vi "NI_SAT_TEST_20150519_EXP_V2.vi"() -> ()   [LabVIEW 2013]
uses:
  <instrlib>/niFgen/niFgen.llb/niFgen Waveform Type.ctl
  <instrlib>/niFgen/niFgen.llb/niFgen Output Impedance.ctl
  <vilib>/Waveform/WDTOps.llb/WDT Append Waveforms DBL.vi
panel:
  out "Tabs 1 Through # Used":i32
  in  "Tab Control 3":T1(tab)
  out "Tab Control 2":T1(tab)
  out "Waveform Graph 1":waveform(dbl)(graph)
  out "Waveform Graph 2":waveform(dbl)(graph)
  out "Waveform Graph 3":waveform(dbl)(graph)
  out "Waveform Graph 4":waveform(dbl)(graph)
  out "Waveform Graph 5":waveform(dbl)(graph)
  out "Waveform Graph 6":waveform(dbl)(graph)
  out "Waveform Graph 7":waveform(dbl)(graph)
  out "Waveform Graph 8":waveform(dbl)(graph)
  out "Waveform Graph 9":waveform(dbl)(graph)
  out "Waveform Graph 10":waveform(dbl)(graph)
  out "Waveform Graph 11":waveform(dbl)(graph)
  out "Waveform Graph 12":waveform(dbl)(graph)
  out "Waveform Graph 13":waveform(dbl)(graph)
  out "Waveform Graph 14":waveform(dbl)(graph)
  out "Waveform Graph 15":waveform(dbl)(graph)
  out "Waveform Graph 16":waveform(dbl)(graph)
  out "Waveform Graph 17":waveform(dbl)(graph)
  out "Waveform Graph 18":waveform(dbl)(graph)
  out "Waveform Graph 19":waveform(dbl)(graph)
  out "Waveform Graph 20":waveform(dbl)(graph)
  out "Diff in Methods before call DMM vi and before read Wave Data (SEC)":dbl
  out "Total Elapsed Time (ms)":u32
  out "TotalElapsed Time (Sec)":dbl
  out "Waveform Graph":waveform(dbl)(graph)
  in  "Output Voltage Division":i32
  in  "Highest Output Voltage [Volts]":i32 min=-200 max=200 step=20
  in  "Rate":dbl=10.0 caption="Rate (Samples/Sec)" format="%.2f"
  in  "Waveform Points":i32=101 caption="Samples"
  in  "Function Generator Name":refnum<k15>="PXI1Slot2"
  # "Please Enter Output Voltage\nwith the desired sign. Be it positive\nor negative. Program will divide 200 and then negate, due to gain of 200 and inversion of input by amplifier"
  # "ENJOY PETER, still could use tweeking to make it run smoother and prevent more user error. Good Morning"
  # "DO NOT RAISE ABOVE 600V on TELFON MASK!!!!!!\nDO NOT RAISE ABOVE 400V on REGULAR MASK!!!"
  # "Output voltage comes from the VOLTAGE MONITOR (VM) from the amplifier with (1V VM/200V AMP)"
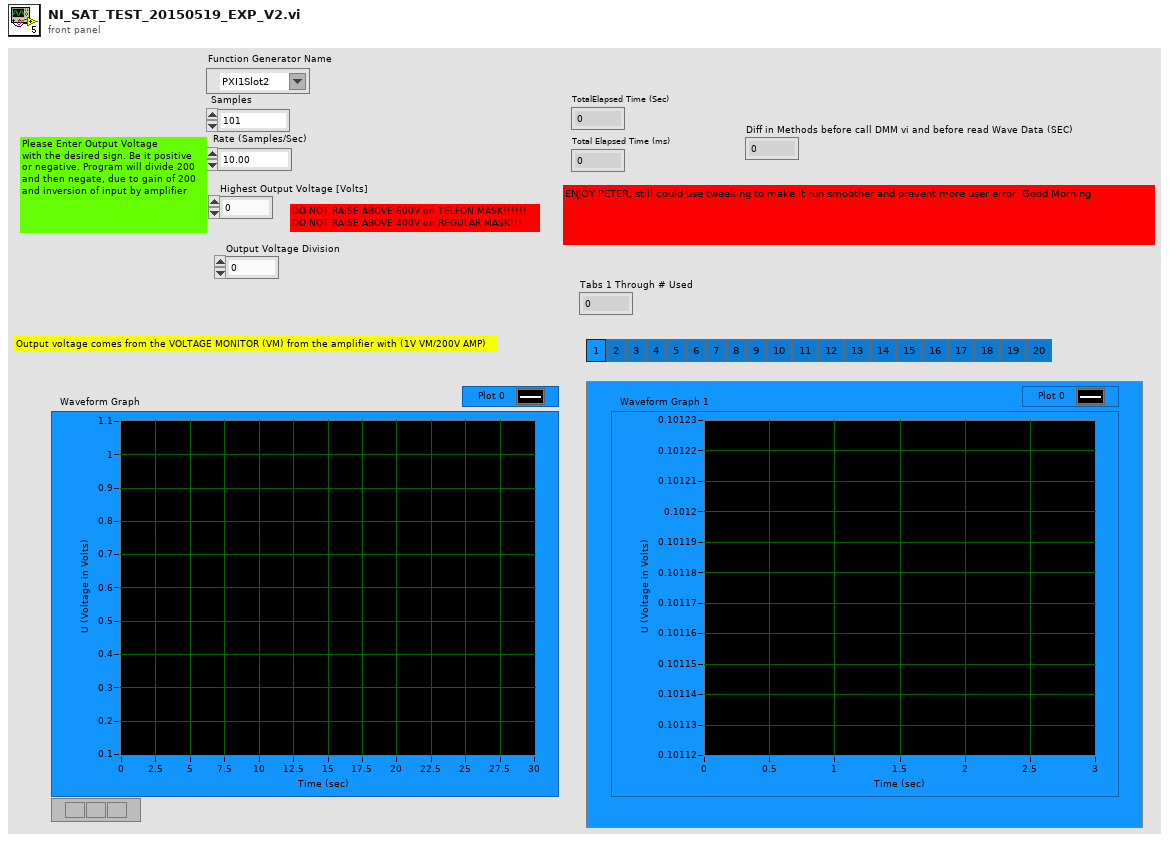
[diagram p1: front panel]
types:
  T1 = enum32{"1", "2", "3", "4", "5", "6", "7", "8", "9", "10", "11", "12", "13", "14", "15", "16", "17", "18", "19", "20"}
  T2 = enum16{"open", "replace", "create", "open or create", "replace or create", "replace or create with confirmation"}
  T3 = typedef "niFgen Output Impedance.ctl" = i32
  T4 = typedef "niFgen Waveform Type.ctl" = i32
  T5 = cluster{"channel name":string, "waveform":T4, "frequency":dbl, "amplitude":dbl, "start phase":dbl, "y":dbl, "duty cycle high":dbl, "impedance":T3, "load impedance":dbl}
  T6 = cluster{"channel name":string, "waveform":T4, "frequency":dbl, "amplitude":dbl, "start phase":dbl, "y":dbl, "duty cycle high":dbl, "impedance":T3, "load impedance":dbl}[]
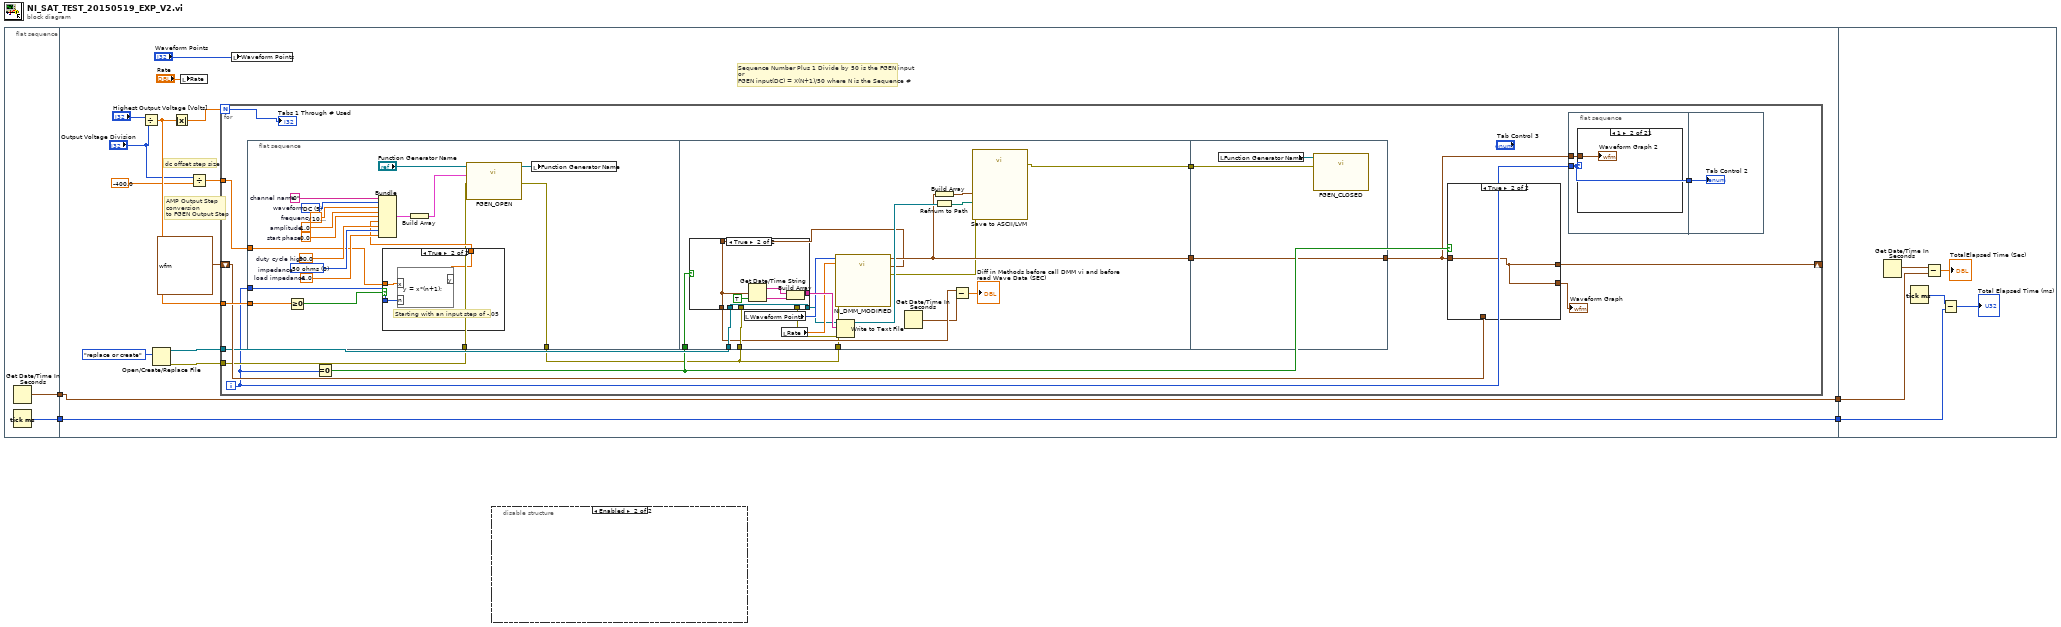
[diagram p0: block diagram]
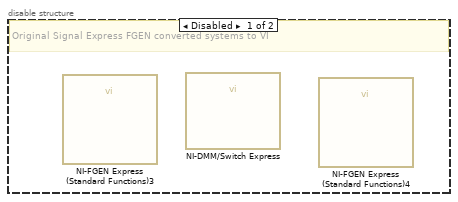
[diagram p2: hidden frame]
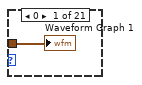
[diagram p3: hidden frame]
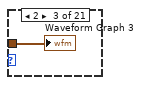
[diagram p4: hidden frame]
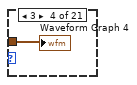
[diagram p5: hidden frame]
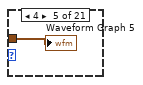
[diagram p6: hidden frame]
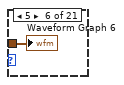
[diagram p7: hidden frame]
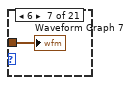
[diagram p8: hidden frame]
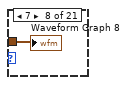
[diagram p9: hidden frame]
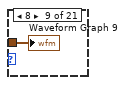
[diagram p10: hidden frame]
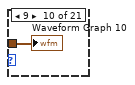
[diagram p11: hidden frame]
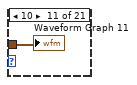
[diagram p12: hidden frame]
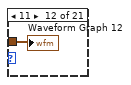
[diagram p13: hidden frame]
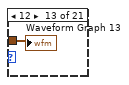
[diagram p14: hidden frame]
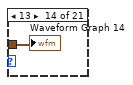
[diagram p15: hidden frame]
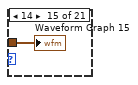
[diagram p16: hidden frame]
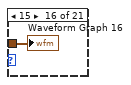
[diagram p17: hidden frame]
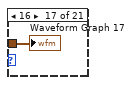
[diagram p18: hidden frame]
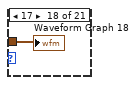
[diagram p19: hidden frame]
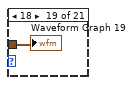
[diagram p20: hidden frame]
diagram:
  n1 = flat-sequence {
    tunnel: [w6] -> w4
    tunnel: [w5] -> w3
    tunnel: w4 -> [w12]
    tunnel: w3 -> [w11]
    tunnel: [w12] -> w2
    tunnel: [w11] -> w1
    tunnel: w2 -> [w129]
    tunnel: w1 -> [w128]
    frame #0 {
      n2 = Get Date/Time In Seconds() -> (seconds since 1Jan1904=w6:timestamp)
      n3 = Tick Count (ms)() -> (millisecond timer value=w5:u32)
    }
    frame #1 {
      # "AMP Output Step\nconversion\nto FGEN Output Step"
      # "dc offset step size"
      # "Sequence Number Plus 1 Divide by 50 is the FGEN input\nor\nFGEN input(DC) = X(N+1)/50 where N is the Sequence #"
      n4 = Divide(x="Highest Output Voltage [Volts]", y="Output Voltage Division") -> (x/y=w10:dbl)
      n5 = Open/Create/Replace File(operation (0:open)=T2."replace or create") -> (refnum out=w20:refnum<file>, error out=w19:errorcluster)  [unwired: 5 in, 1 out]
      n6 = Absolute Value(x=w10) -> (abs(x)=w14:dbl)
      n7 = local write "Rate"("Rate") -> ()
      n8 = Divide(x="Output Voltage Division", y=-400.0) -> (x/y=w9:dbl)
      n9 = for {
        N: w14 -> [w23]
        tunnel: w20 -> [w31]
        tunnel: w19 -> [w28]
        tunnel: w10 -> [w34]
        shift-right: [w26] -> _
        shift-left: waveform(dbl) {"t0"=timestamp(0 s since 1904-01-01), "dt"=1.0, "Y"=[]} ("Waveform Data") -> [w33]
        tunnel: w9 -> [w21]
        i -> [w24]
        n10 = flat-sequence {
          tunnel: w24 -> [w71]
          tunnel: w34 -> [w68]
          tunnel: w28 -> [w65]
          tunnel: [w64] -> w27
          tunnel: w21 -> [w63]
          tunnel: [w102] -> w35
          tunnel: w30 -> [w99]
          tunnel: w31 -> [w98]
          tunnel: w27 -> [w96]
          tunnel: [w93] -> w29
          tunnel: w27 -> [w89]
          tunnel: w35 -> [w126]
          tunnel: [w126] -> w25
          tunnel: w29 -> [w125]
          frame #0 {
            w72 = -1.0  # load impedance
            w73 = T3 0 items=["50 ohms", "75 ohms", "1 mega ohm"]  # impedance
            w74 = 50.0  # duty cycle high
            w75 = 0.0  # start phase
            w76 = 1.0  # amplitude
            w77 = 1000000.0  # frequency
            w78 = T4 5 items=["Sine", "Square", "Triangle", "Ramp Up", "Ramp Down", "DC", "Noise", "User"]  # waveform
            w79 = "0"  # channel name
            n11 = Greater Or Equal To 0?(x=w68) -> (x >= 0?=w67:bool)
            n12 = case shown="True" w67 {
              tunnel: w71 -> [w83 w87]
              tunnel: w63 -> [w84 w86]
              tunnel: [w82 w85] -> w66
              frame False {
                # "Starting with an input step of .05"
                # "Negative Output"
                n13 = formula code="y = -x*(n+1);"("x"=w84, "n"=w83) -> ("y"=w82:dbl)
              }
              frame True {
                # "Starting with an input step of -.05"
                n14 = formula code="y = x*(n+1);"("x"=w86, "n"=w87) -> ("y"=w85:dbl)
              }
            }
            n15 = Bundle("channel name"=w79, "waveform"=w78, "frequency"=w77, "amplitude"=w76, "start phase"=w75, "y"=w66, "duty cycle high"=w74, "impedance"=w73, "load impedance"=w72) -> (w70:T5)  [unwired: 1 in]
            n16 = Build Array(w70) -> (w69:T6)
            n17 = call "FGEN_OPEN.vi"("error in"=w65, "channel parameters"=w69, "resource name"="Function Generator Name") -> ("error out"=w64:errorcluster, "Instrument Handle Out"=w81:refnum<k15>)  [unwired: 7 in]
            n18 = local write "Function Generator Name"(w81) -> ()
          }
          frame #1 {
            n19 = local read "Waveform Points"() -> (w101:i32)
            n20 = local read "Rate"() -> (w100:dbl)
            n21 = call "NI_DMM_MODIFIED.vi"("Waveform Points"=w101, "Rate"=w100, "error in"=w89) -> ("Waveform Data"=w102:waveform(dbl), "current time"=w90:timestamp, "error out"=w94:errorcluster)  [unwired: 14 in]
            n22 = case shown="True" w99 {
              tunnel: [w113 w121] -> w106
              tunnel: w98 -> [w111 w120]
              tunnel: [w109 w120] -> w97
              tunnel: w96 -> [w110 w119]
              tunnel: [w108 w119] -> w95
              tunnel: [w107 w118] -> w92
              tunnel: w90 -> [w107 w118]
              frame False {
                n23 = Get Date/Time String(seconds (now)=w107, want seconds? (F)=TRUE) -> (date string=w116:string, time string=w115:string)  [unwired: 1 in]
                n24 = Set File Position(refnum=w111, from (0:start)=enum16{"start", "end", "current"}."end", error in=w110) -> (refnum out=w109:refnum<file>, error out=w108:errorcluster)  [unwired: 1 in]
                n25 = Build Array("" ("element"), w116, w115) -> (w113:string[])
              }
              frame True {
                n26 = Get Date/Time String(seconds (now)=w118, want seconds? (F)=TRUE) -> (date string=w123:string, time string=w122:string)  [unwired: 1 in]
                n27 = Build Array(w123, w122) -> (w121:string[])
              }
            }
            n28 = Write to Text File(file (use dialog)=w97, text=w106, error in=w95) -> (refnum out=w105:refnum<file>)  [unwired: 1 in, 2 out]
            n29 = Get Date/Time In Seconds() -> (seconds since 1Jan1904=w88:timestamp)
            n30 = Build Array(w102) -> (w103:waveform(dbl)[])
            n31 = Refnum to Path(1:w105) -> (0:w104:path)
            n32 = Subtract(x=w92, y=w88) -> (x-y=→"Diff in Methods before call DMM vi and before read Wave Data (SEC)":dbl)
            n33 = call "Save to ASCII/LVM"("signals in"=w103, "File Path"=w104, "error in"=w94) -> ("error out"=w93:errorcluster)  [unwired: 16 in]
          }
          frame #2 {
            n34 = local read "Function Generator Name"() -> (w127:refnum<k15>)
            n35 = call "FGEN_CLOSED.vi"("error in"=w125, "instrument handle"=w127) -> ()  [unwired: 9 in, 1 out]
          }
        }
        n36 = Equal To 0?(x=w24) -> (x = 0?=w30:bool)
        n37 = case shown="True" w30 {
          tunnel: w25 -> [w59 w62]
          tunnel: [w60 w62] -> w26
          tunnel: w33 -> [w61 _]
          tunnel: [w60 w62] -> w32
          frame False {
            n38 = call-poly <vilib>:"Append Waveforms.vi"("waveform B"=w59, "waveform A"=w61) -> ("waveform out"=w60:waveform(dbl))  [unwired: 8 in, 1 out]
          }
          frame True {
          }
        }
        "Waveform Graph" <- w32
        n39 = flat-sequence {
          tunnel: w25 -> [w37]
          tunnel: w24 -> [w36]
          tunnel: [w36] -> w22
          tunnel: w22 -> [w58]
          frame #0 {
            n40 = case shown="1" w36 {
              tunnel: w37 -> [w38 w39 w40 w41 w42 w43 w44 w45 w46 w47 w48 w49 w50 w51 w52 w53 w54 w55 w56 w57 _]
              frame 0 {
                "Waveform Graph 1" <- w38
              }
              frame 1 {
                "Waveform Graph 2" <- w39
              }
              frame 2 {
                "Waveform Graph 3" <- w40
              }
              frame 3 {
                "Waveform Graph 4" <- w41
              }
              frame 4 {
                "Waveform Graph 5" <- w42
              }
              frame 5 {
                "Waveform Graph 6" <- w43
              }
              frame 6 {
                "Waveform Graph 7" <- w44
              }
              frame 7 {
                "Waveform Graph 8" <- w45
              }
              frame 8 {
                "Waveform Graph 9" <- w46
              }
              frame 9 {
                "Waveform Graph 10" <- w47
              }
              frame 10 {
                "Waveform Graph 11" <- w48
              }
              frame 11 {
                "Waveform Graph 12" <- w49
              }
              frame 12 {
                "Waveform Graph 13" <- w50
              }
              frame 13 {
                "Waveform Graph 14" <- w51
              }
              frame 14 {
                "Waveform Graph 15" <- w52
              }
              frame 15 {
                "Waveform Graph 16" <- w53
              }
              frame 16 {
                "Waveform Graph 17" <- w54
              }
              frame 17 {
                "Waveform Graph 18" <- w55
              }
              frame 18 {
                "Waveform Graph 19" <- w56
              }
              frame 19 {
                "Waveform Graph 20" <- w57
              }
              frame 20, Default {
              }
            }
          }
          frame #1 {
            "Tab Control 2" <- w58
          }
        }
        "Tabs 1 Through # Used" <- w23
      }
      n41 = local write "Waveform Points"("Waveform Points") -> ()
    }
    frame #2 {
      n42 = Get Date/Time In Seconds() -> (seconds since 1Jan1904=w130:timestamp)
      n43 = Tick Count (ms)() -> (millisecond timer value=w132:u32)
      n44 = Subtract(x=w130, y=w129) -> (x-y=→"TotalElapsed Time (Sec)":dbl)
      n45 = Subtract(x=w132, y=w128) -> (x-y=→"Total Elapsed Time (ms)":u32)
    }
  }
  n46 = disable-structure shown="Enabled" {
    frame Disabled {
      # "Original Signal Express FGEN converted systems to VI"
      n47 = call "NI-FGEN Express (Standard Functions)3"() -> ()  [unwired: 11 in, 1 out]
      n48 = call "NI-DMM/Switch Express"() -> ()  [unwired: 17 in, 3 out]
      n49 = call "NI-FGEN Express (Standard Functions)4"() -> ()  [unwired: 11 in, 1 out]
    }
    frame Enabled {
    }
  }
